vi "Can Stop.vi"(7 "Actor in":refnum<class "Actor.lvclass">, 8 "Error in":errorcluster, 10 "From Msg Event":bool) -> (0 "Error out":errorcluster, 2 "Stop":bool, 5 "Actor out":refnum<class "Actor.lvclass">)   [LabVIEW 2025, in "jettl.lvlib" / "Actor.lvlib"]
uses:
  Actor.lvlib
  Actor/Actor.lvclass
  Stop Msg/Call.vi
  Stop Msg/Stop Msg.lvlib
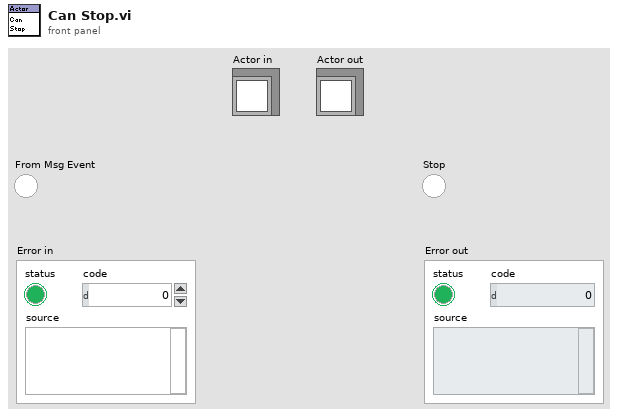
[diagram p1: front panel]
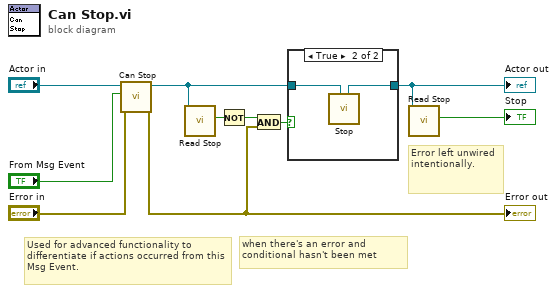
[diagram p0: block diagram]
diagram:
  # "Error left unwired intentionally."
  # "when there's an error and conditional hasn't been met"
  # "Used for advanced functionality to differentiate if actions occurred from this Msg Event."
  n1 = call-dynamic "Can Stop.vi"("Error in"="Error in", "From Msg Event"="From Msg Event", "Actor in"="Actor in") -> ("Error out"=w3:errorcluster, "Actor out"=w4:refnum<class "Actor.lvclass">)  [unwired: 7 in]
  "Error out" <- w3
  n2 = call-dynamic "Read Stop.vi"("Actor in"=w4) -> ("Stop"=w5:bool)  [unwired: 10 in]
  n3 = Not(x=w5) -> (.not. x?=w7:bool)
  n4 = And(x=w7, y=w3) -> (x .and. y?=w6:bool)
  n5 = case shown="True" w6 {
    tunnel: [w11 w12] -> w2
    tunnel: w4 -> [w11 w13]
    frame False {
    }
    frame True {
      n6 = call-poly "Stop.vi"("Actor in"=w13) -> ("Actor out"=w12:refnum<class "Actor.lvclass">)  [unwired: 9 in, 1 out]
    }
  }
  "Actor out" <- w2
  n7 = call-dynamic "Read Stop.vi"("Actor in"=w2) -> ("Stop"=→"Stop":bool)  [unwired: 10 in]
